vi "DecodeHeader.vi"(8 "error in (no error)":errorcluster, 11 "Header file path":path=path "C:/Users/Andrzej/Desktop/Dropbox/SharedForDADMProj/sygnały/100.hea") -> (0 "error out":errorcluster, 1 "Segments Spec Info":T1[](array[typedef]), 2 "Signals Specs Info":T2[](array[typedef]), 3 "Record Line Info":T3, 4 "Info Strings":string[](array[string]), 5 "Comment Lines":string[](array[string]))   [LabVIEW 2012]
doc: "Reads and decodes information contained in a header (.hea) file of a Physionet record. <b>Record Line Info</b> is a cluster containing information common for all signals. <b>Signals Spec Info</b> is an array of clusters with information about all signals in a record. <b>Comment Lines</b> is an array of strings with all comment lines from the .hea file. <b>Info Strings</b> contains all the comment lines from the end of the file."
uses:
  #TD_RecordLineInfo.ctl
  #TD_SignalSpecInfo.ctl
  #TD_SegmentSpecInfo.ctl
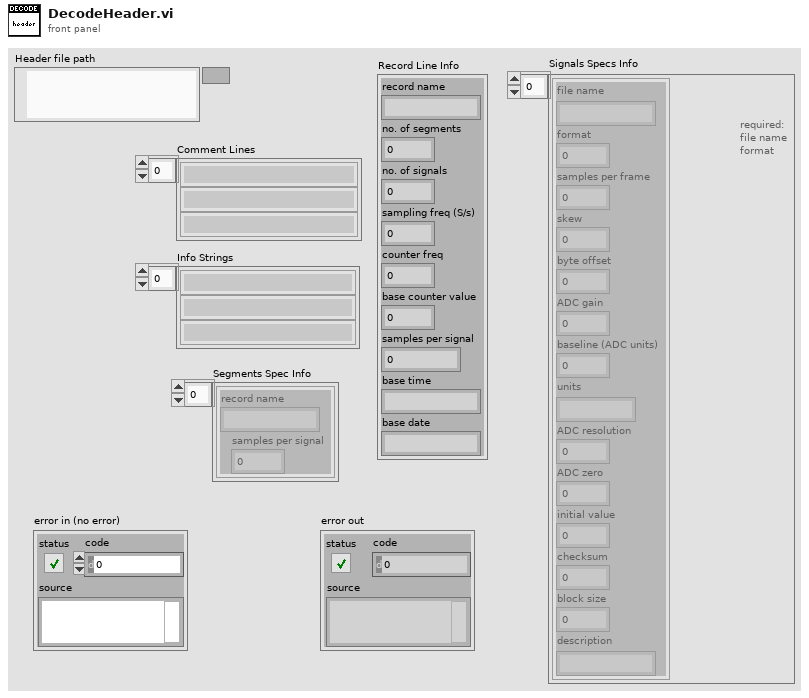
[diagram p1: front panel]
types:
  T1 = typedef "#TD_SegmentSpecInfo.ctl" = cluster{"record name":string, "samples per signal":i32}
  T2 = typedef "#TD_SignalSpecInfo.ctl" = cluster{"file name":string, "format":i32, "samples per frame":i32, "skew":i32, "byte offset":i32, "ADC gain":dbl, "baseline (ADC units)":i16, "units":string, "ADC resolution":i16, "ADC zero":i16, "initial value":i16, "checksum":i16, "block size":i32, "description":string}
  T3 = typedef "#TD_RecordLineInfo.ctl" = cluster{"record name":string, "no. of segments":i32, "no. of signals":i32, "sampling freq (S/s)":dbl, "counter freq":dbl, "base counter value":dbl, "samples per signal":i32, "base time":string, "base date":string}
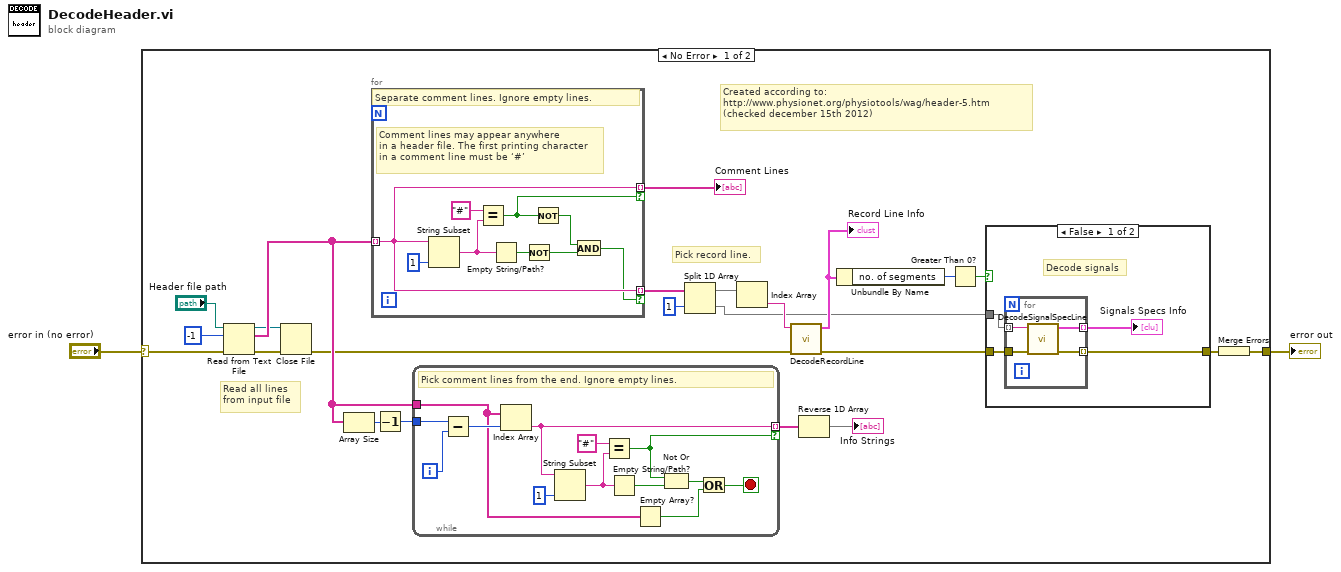
[diagram p0: block diagram]
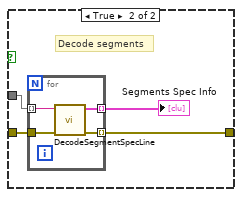
[diagram p2: hidden frame]
diagram:
  n1 = case shown="No Error" "error in (no error)" {
    selector: "error in (no error)" -> [w7 w64]
    tunnel: [w3 w64] -> w1
    frame No Error {
      # "Created according to:\nhttp://www.physionet.org/physiotools/wag/header-5.htm\n(checked december 15th 2012)"
      # "Pick record line."
      # "Read all lines\nfrom input file"
      n2 = Read from Text File(file (use dialog)="Header file path", count=-1, error in=w7) -> (refnum out=w8:refnum<file>, text=w10:string[], error out=w9:errorcluster)  [unwired: 1 in, 1 out]
      n3 = Close File(refnum=w8, error in=w9) -> (error out=w6:errorcluster)  [unwired: 1 out]
      n4 = Array Size(array=w10) -> (size(s)=w17:i32)
      n5 = for {
        tunnel: w10 -> [w61] mode=indexing
        tunnel: [w61] -> w24 mode=indexing if=w55
        tunnel: [w61] -> w23 mode=indexing if=w56
        # "Comment lines may appear anywhere \nin a header file. The first printing character\nin a comment line must be ‘#’"
        # "Separate comment lines. Ignore empty lines."
        n6 = String Subset(string=w61, length (rest)=1 ("length (rest)")) -> (substring=w60:string)  [unwired: 1 in]
        n7 = Equal?(x="#", y=w60) -> (x = y?=w55:bool)
        n8 = Empty String/Path?(string/path=w60) -> (empty?=w59:bool)
        n9 = Not(x=w59) -> (.not. x?=w57:bool)
        n10 = Not(x=w55) -> (.not. x?=w58:bool)
        n11 = And(x=w58, y=w57) -> (x .and. y?=w56:bool)
      }
      "Comment Lines" <- w24
      n12 = Decrement(x=w17) -> (x-1=w16:i32)
      n13 = while {
        tunnel: [w47] -> w15 mode=indexing if=w46
        tunnel: w10 -> [w45]
        tunnel: w16 -> [w49]
        i -> [w50]
        stop <- w42 stop-if-true
        # "Pick comment lines from the end. Ignore empty lines."
        n14 = Subtract(x=w49, y=w50) -> (x-y=w48:i32)
        n15 = Index Array(array=w45, index=w48) -> (element=w47:string)
        n16 = String Subset(string=w47, length (rest)=1 ("length (rest)")) -> (substring=w54:string)  [unwired: 1 in]
        n17 = Equal?(x="#", y=w54) -> (x = y?=w46:bool)
        n18 = Empty String/Path?(string/path=w54) -> (empty?=w51:bool)
        n19 = Empty Array?(array=w45) -> (empty?=w43:bool)
        n20 = Not Or(1:w51, 2:w46) -> (0:w44:bool)
        n21 = Or(x=w44, y=w43) -> (x .or. y?=w42:bool)
      }
      n22 = Split 1D Array(array=w23, index=1) -> (first subarray=w21:string[], second subarray=w11:string[])
      n23 = Index Array(array=w21) -> (element=w19:string)  [unwired: 1 in]
      n24 = call "DecodeRecordLine.vi"("error in (no error)"=w6, "Record Line"=w19) -> ("error out"=w5:errorcluster, "Record Line info"=w14:T3)  [unwired: 8 in]
      "Record Line Info" <- w14
      n25 = Reverse 1D Array(array=w15) -> (reversed array=→"Info Strings":string[])
      n26 = Unbundle By Name(w14) -> ("no. of segments"=w13:i32)
      n27 = Greater Than 0?(x=w13) -> (x > 0?=w12:bool)
      n28 = case shown="False" w12 {
        tunnel: w11 -> [w29 w37]
        tunnel: w5 -> [w28 w36]
        tunnel: [w27 w35] -> w4
        frame False {
          # "Decode signals"
          n29 = for {
            tunnel: w29 -> [w33] mode=indexing
            tunnel: [w32] -> w26 mode=indexing
            tunnel: w28 -> [w31]
            tunnel: [w30] -> w27 mode=indexing
            n30 = call "DecodeSignalSpecLine.vi"("error in (no error)"=w31, "Signal Spec Line"=w33) -> ("error out"=w30:errorcluster, "Signal Spec Info"=w32:T2)  [unwired: 8 in]
          }
          "Signals Specs Info" <- w26
        }
        frame True {
          # "Decode segments"
          n31 = for {
            tunnel: w37 -> [w40] mode=indexing
            tunnel: [w41] -> w34 mode=indexing
            tunnel: w36 -> [w39]
            tunnel: [w38] -> w35 mode=indexing
            n32 = call "DecodeSegmentSpecLine.vi"("error in (no error)"=w39, "Segment Spec Line"=w40) -> ("error out"=w38:errorcluster, "Segment Spec Info"=w41:T1)  [unwired: 8 in]
          }
          "Segments Spec Info" <- w34
        }
      }
      n33 = Merge Errors(w4) -> (w3:errorcluster)
    }
    frame Error {
    }
  }
  "error out" <- w1
